vi "Teleop.vi"(10 "Match Info":T1={"Autonomous Elapsed Seconds"=0.0, "TeleOp Elapsed Seconds"=0.0, "Disabled Elapsed Seconds"=0.0, "Visited Autonomous"=FALSE, "Visited TeleOp"=FALSE, "Visited Disabled"=FALSE, "Autonomous Settings"={"Autonomous Style"=enum."Independent", "VI Refnum"=refnum}}, 11 "Call Context":T2) -> ()   [LabVIEW 2012]
doc: "This VI is called for each TeleOp packet received from the DS where the robot is not disabled. It is often used to read from the joysticks and update I/O or to update setpoints for timed control loops. It should complete and return within 20 milliseconds or it may miss DS packets."
uses:
  <vilib>/Rock Robotics/WPI/DriverStation/WPI_DriverStationDerivedRobotMode.ctl
  <vilib>/Rock Robotics/WPI/DriverStation/WPI_DriverStationMatch Info.ctl
  <vilib>/Rock Robotics/WPI/Relay/WPI_RelayValue.ctl
  Robot Global Data.vi
  <vilib>/Rock Robotics/WPI/Joystick/WPI_JoystickGetSetRefNum.vi
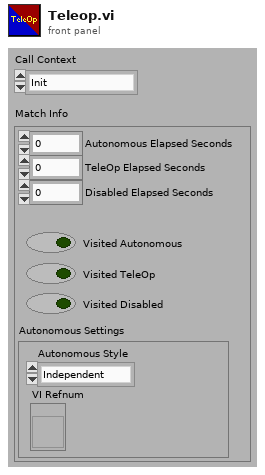
[diagram p1: front panel]
types:
  T1 = typedef "WPI_DriverStationMatch Info.ctl" = cluster{"Autonomous Elapsed Seconds":dbl, "TeleOp Elapsed Seconds":dbl, "Disabled Elapsed Seconds":dbl, "Visited Autonomous":bool, "Visited TeleOp":bool, "Visited Disabled":bool, "Autonomous Settings":cluster{"Autonomous Style":enum16{"Iterative", "Independent"}, "VI Refnum":refnum<vi>}}
  T2 = typedef "WPI_DriverStationDerivedRobotMode.ctl" = enum16{"Init", "Execute", "Stop"}
  T3 = typedef "WPI_RelayValue.ctl" = enum16{"Off", "On", "Forward", "Reverse"}
  T4 = typedef "WPI_JoystickDevRef.ctl" = cluster{"Device":T5}
  T5 = typedef "WPI_JoystickDeviceEnum.ctl" = enum16{"USB 1", "USB 2", "USB 3", "USB 4", "Kinect 1", "Kinect 2"}
  T6 = cluster{"axis 1 (x)":dbl, "axis 2 (y)":dbl, "axis 3 (throttle)":dbl, "axis 4":dbl, "axis 5":dbl, "axis 6":dbl}
  T7 = typedef "WPI_RelayDevRef.ctl" = cluster{"DevStatus":errorcluster, "Relay Channel":T8, "Digital Module":T9, "Relay Direction":T10}
  T8 = typedef "FPGA_DIORelayChannel.ctl" = enum8{"Relay 1", "Relay 2", "Relay 3", "Relay 4", "Relay 5", "Relay 6", "Relay 7", "Relay 8", "Invalid"}
  T9 = typedef "FPGA_TypedefDigitalModule.ctl" = enum16{"Digital Module 1", "Digital Module 2"}
  T10 = typedef "WPI_RelayDirection.ctl" = enum16{"Both directions", "Forward only", "Reverse only"}
  T11 = cluster{"Driver Station Digital Input (1-8)[0]":bool, "Driver Station Digital Input (1-8)[1]":bool, "Driver Station Digital Input (1-8)[2]":bool, "Driver Station Digital Input (1-8)[3]":bool, "Driver Station Digital Input (1-8)[4]":bool, "Driver Station Digital Input (1-8)[5]":bool, "Driver Station Digital Input (1-8)[6]":bool, "Driver Station Digital Input (1-8)[7]":bool, "Driver Station Digital Input (1-8)[8]":bool}
  T12 = cluster{"Shifting":cluster{"Right Servo High":dbl, "Right Servo Low":dbl, "Left Servo High":dbl, "Left Servo Low":dbl}, "Breaking":cluster{"Coast Position":dbl, "Break Position":dbl}}
  T13 = typedef "WPI_JoystickButtonState.ctl" = cluster{"Button 1":bool, "Button 2":bool, "Button 3":bool, "Button 4":bool, "Button 5":bool, "Button 6":bool, "Button 7":bool, "Button 8":bool, "Button 9":bool, "Button 10":bool, "Button 11":bool, "Button 12":bool}
  T14 = typedef "WPI_MotorControlDeviceRef.ctl" = cluster{"DeviceStatus":errorcluster, "Type":enum16{"PWM", "CAN"}, "PWM":cluster{"Digital Module":T9, "PWM Channel":T15, "DeadBand":T16}, "CAN":cluster{"Device Number":u8, "Control Mode":T17, "Semaphore":T18, "Max Vout":dbl}, "Invert":bool, "TransformRef":T19, "InvTransformRef":T19}
  T15 = typedef "FPGA_DIOPWMChannel.ctl" = enum8{"PWM 1", "PWM 2", "PWM 3", "PWM 4", "PWM 5", "PWM 6", "PWM 7", "PWM 8", "PWM 9", "PWM 10", "Invalid"}
  T16 = typedef "WPI_PWMDeadband.ctl" = cluster{"Name":string, "maxPositivePwm":i32, "minPositivePwm":i32, "centerPwm":i32, "maxNegativePwm":i32, "minNegativePwm":i32, "angularRange":u16}
  T17 = typedef "WPI_CANJaguar_ControlMode.ctl" = enum8{"Percent VBus", "Current", "Speed", "Position", "Voltage"}
  T18 = typedef "Semaphore RefNum" = refnum<k1>
  T19 = typedef "WPI_PWMTransform_ConPane.ctl" = refnum<vi>
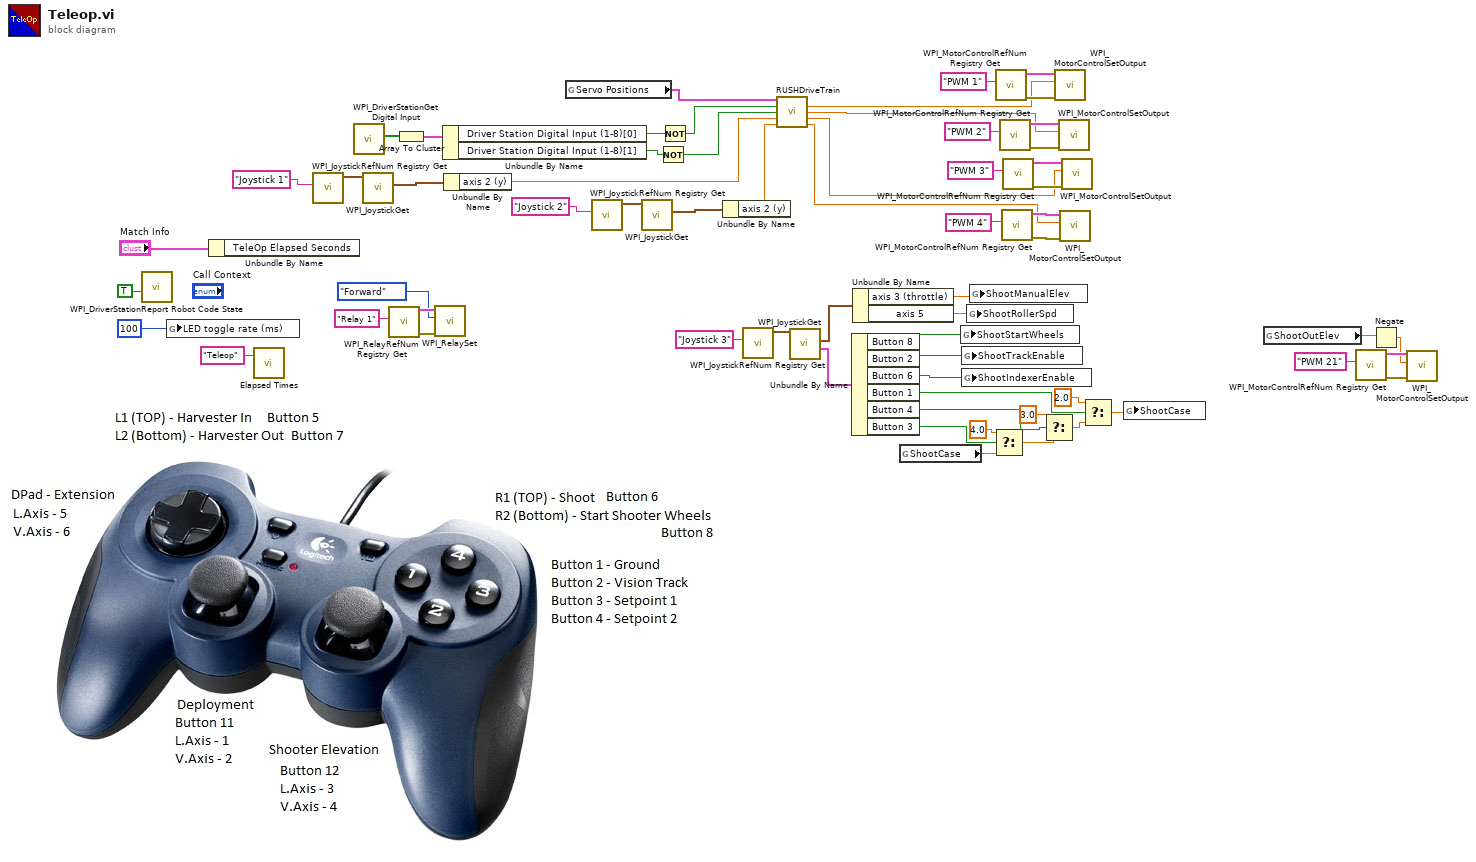
[diagram p0: block diagram]
diagram:
  n1 = call <vilib>:"WPI_DriverStationReport Robot Code State.vi"("TeleOp"=TRUE ("Autonomous")) -> ()  [unwired: 10 in, 1 out]
  n2 = global write "Robot Global Data.vi" "LED toggle rate (ms)"(u32 100 ("LED ms toggle rate")) -> ()
  n3 = Unbundle By Name("Match Info") -> ()  [unwired: 1 out]
  n4 = call "Elapsed Times.vi"("Call Name"="Teleop") -> ()  [unwired: 2 in, 1 out]
  n5 = call <vilib>:"WPI_JoystickRefNum Registry Get.vi"("refnum name"="Joystick 1") -> ("JoystickDevRef"=w46:T4)  [unwired: 1 in, 9 out]
  n6 = call <vilib>:"WPI_DriverStationGet Digital Input.vi"() -> ("Driver Station Digital Input (1-8)"=w41:bool[])  [unwired: 11 in]
  n7 = call <vilib>:"WPI_JoystickGet.vi"("JoystickDevRef"=w46) -> ("Axes"=w45:T6)  [unwired: 1 in, 5 out]
  n8 = call <vilib>:"WPI_RelayRefNum Registry Get.vi"("refnum name"="Relay 1") -> ("error out"=w57:errorcluster, "RelayDevRef"=w59:T7)  [unwired: 9 in]
  n9 = Array To Cluster(array=w41) -> (cluster=w40:T11)
  n10 = call <vilib>:"WPI_RelaySet.vi"("error in (no error)"=w57, "RelayValue"=WPI_RelayValue."Forward", "RelayDevRef"=w59) -> ()  [unwired: 7 in, 2 out]
  n11 = Unbundle By Name(w40) -> ("Driver Station Digital Input (1-8)[0]"=w39:bool, "Driver Station Digital Input (1-8)[1]"=w38:bool)
  n12 = Unbundle By Name(w45) -> ("axis 2 (y)"=w35:dbl)
  n13 = global read "Robot Global Data.vi" "Servo Positions"() -> (w33:T12)
  n14 = call <vilib>:"WPI_JoystickRefNum Registry Get.vi"("refnum name"="Joystick 2") -> ("JoystickDevRef"=w43:T4)  [unwired: 1 in, 9 out]
  n15 = call <vilib>:"WPI_JoystickGet.vi"("JoystickDevRef"=w43) -> ("Axes"=w44:T6)  [unwired: 1 in, 5 out]
  n16 = Not(x=w38) -> (.not. x?=w36:bool)
  n17 = Not(x=w39) -> (.not. x?=w37:bool)
  n18 = Unbundle By Name(w44) -> ("axis 2 (y)"=w34:dbl)
  n19 = call <vilib>:"WPI_JoystickRefNum Registry Get.vi"("refnum name"="Joystick 3") -> ("JoystickDevRef"=w55:T4)  [unwired: 9 in, 1 out]
  n20 = call "RUSHDriveTrain.vi"("Servo Positions"=w33, "Low Gear + Brake"=w37, "Low Gear"=w36, "LeftJoystick"=w35, "RightJoystick"=w34) -> ("Left Drive"=w20:dbl, "Right Drive"=w19:dbl, "Left Servo"=w18:dbl, "Right Servo"=w1:dbl)  [unwired: 6 in, 1 out]
  n21 = call <vilib>:"WPI_JoystickGet.vi"("JoystickDevRef"=w55) -> ("Buttons"=w53:T13, "Axes"=w52:T6)  [unwired: 4 in, 1 out]
  n22 = Unbundle By Name(w53) -> ("Button 8"=w49:bool, "Button 2"=w50:bool, "Button 6"=w51:bool, "Button 1"=w16:bool, "Button 4"=w14:bool, "Button 3"=w13:bool)
  n23 = Unbundle By Name(w52) -> ("axis 3 (throttle)"=w48:dbl, "axis 5"=w17:dbl)
  n24 = global read "Robot Global Data.vi" "ShootCase"() -> (w8:dbl)
  n25 = global write "Robot Global Data.vi" "ShootStartWheels"(w49) -> ()
  n26 = global write "Robot Global Data.vi" "ShootTrackEnable"(w50) -> ()
  n27 = global write "Robot Global Data.vi" "ShootIndexerEnable"(w51) -> ()
  n28 = global write "Robot Global Data.vi" "ShootRollerSpd"(w17) -> ()
  n29 = global write "Robot Global Data.vi" "ShootManualElev"(w48) -> ()
  n30 = Select(t=4.0, s=w13, f=w8) -> (s? t:f=w12:dbl)
  n31 = call <vilib>:"WPI_MotorControlRefNum Registry Get.vi"("refnum name"="PWM 1") -> ("error out"=w21:errorcluster, "MotorControlDevRef"=w22:T14)  [unwired: 9 in]
  n32 = call <vilib>:"WPI_MotorControlRefNum Registry Get.vi"("refnum name"="PWM 2") -> ("error out"=w26:errorcluster, "MotorControlDevRef"=w25:T14)  [unwired: 9 in]
  n33 = call <vilib>:"WPI_MotorControlRefNum Registry Get.vi"("refnum name"="PWM 4") -> ("error out"=w32:errorcluster, "MotorControlDevRef"=w31:T14)  [unwired: 9 in]
  n34 = call <vilib>:"WPI_MotorControlRefNum Registry Get.vi"("refnum name"="PWM 3") -> ("error out"=w27:errorcluster, "MotorControlDevRef"=w28:T14)  [unwired: 9 in]
  n35 = Select(t=3.0, s=w14, f=w12) -> (s? t:f=w10:dbl)
  n36 = call <vilib>:"WPI_MotorControlSetOutput.vi"("error in (no error)"=w21, "Output"=w20, "MotorControlDevRef"=w22) -> ()  [unwired: 6 in, 3 out]
  n37 = call <vilib>:"WPI_MotorControlSetOutput.vi"("error in (no error)"=w26, "Output"=w19, "MotorControlDevRef"=w25) -> ()  [unwired: 6 in, 3 out]
  n38 = call <vilib>:"WPI_MotorControlSetOutput.vi"("error in (no error)"=w32, "Output"=w1, "MotorControlDevRef"=w31) -> ()  [unwired: 6 in, 3 out]
  n39 = call <vilib>:"WPI_MotorControlSetOutput.vi"("error in (no error)"=w27, "Output"=w18, "MotorControlDevRef"=w28) -> ()  [unwired: 6 in, 3 out]
  n40 = Select(t=2.0, s=w16, f=w10) -> (s? t:f=w7:dbl)
  n41 = global write "Robot Global Data.vi" "ShootCase"(w7) -> ()
  n42 = global read "Robot Global Data.vi" "ShootOutElev"() -> (w3:dbl)
  n43 = call <vilib>:"WPI_MotorControlRefNum Registry Get.vi"("refnum name"="PWM 21") -> ("error out"=w6:errorcluster, "MotorControlDevRef"=w5:T14)  [unwired: 9 in]
  n44 = Negate(x=w3) -> (-x=w2:dbl)
  n45 = call <vilib>:"WPI_MotorControlSetOutput.vi"("error in (no error)"=w6, "Output"=w2, "MotorControlDevRef"=w5) -> ()  [unwired: 6 in, 3 out]
